vi "AB_Add_Destination_CORE.vi"(8 "error in (no error)":errorcluster, 9 "destination path":path, 10 "destination label":string, 11 "destinations in":refnum<class "AB_Destination.lvclass">[](array[class])) -> (0 "error out":errorcluster, 2 "destination index":i32, 3 "destinations out":refnum<class "AB_Destination.lvclass">[](array[class]))   [LabVIEW 2020]
uses:
  <vilib>/AppBuilder/AB_Classes/Destination/AB_Destination.lvclass
  <vilib>/AppBuilder/AB_Classes/Destination/AB_Destination.ctl
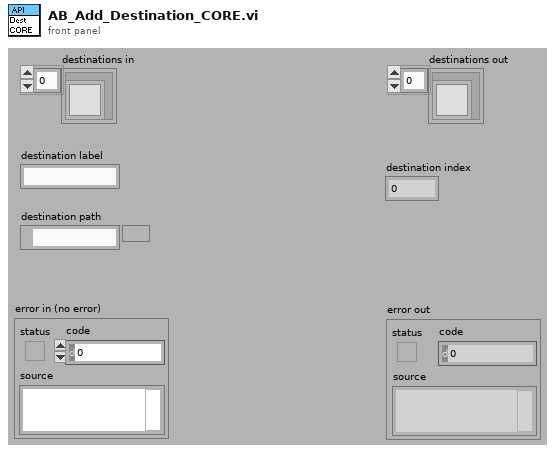
[diagram p1: front panel]
types:
  T1 = typedef "AB_Destination.ctl" = cluster{"destName":string, "path":path, "libraryName":string, "preserveHierarchy":bool, "eng_inBuild":bool, "eng_libraryReference":refnum<vi>, "eng_restictAddToNewLibrary":bool}
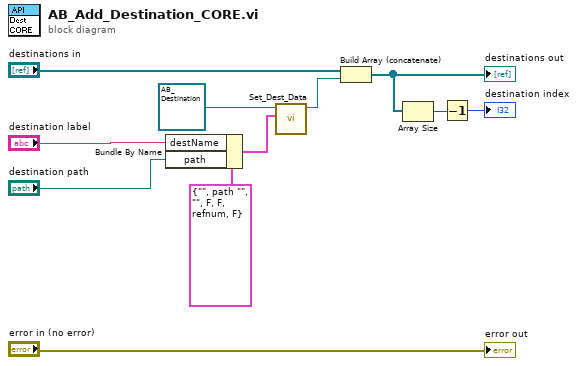
[diagram p0: block diagram]
diagram:
  n1 = Bundle By Name(cluster=T1 {"destName"="", "path"=path "", "libraryName"="", "preserveHierarchy"=FALSE, "eng_inBuild"=FALSE, "eng_libraryReference"=refnum, "eng_restictAddToNewLibrary"=FALSE} ("destName"), "destName"="destination label", "path"="destination path") -> (w9:T1)
  n2 = call <vilib>:"Set_Dest_Data.vi"("destName"=w9, "Class in"=refnum<class "AB_Destination.lvclass"> refnum ("AB_Destination.lvclass")) -> ("Class out"=w10:refnum<class "AB_Destination.lvclass">)  [unwired: 1 in, 8 out]
  n3 = Build Array (concatenate)("destinations in", w10) -> (w3:refnum<class "AB_Destination.lvclass">[])
  "destinations out" <- w3
  n4 = Array Size(array=w3) -> (size(s)=w2:i32)
  n5 = Decrement(x=w2) -> (x-1=→"destination index":i32)
  "error out" <- "error in (no error)"
